vi "Event Structure String Replace Space 5.vi"() -> ()   [LabVIEW 2020]
panel:
  out "length":i32
  in  "String":string
  in  "Stop":bool
  # "Event Structure String : Replace Space"
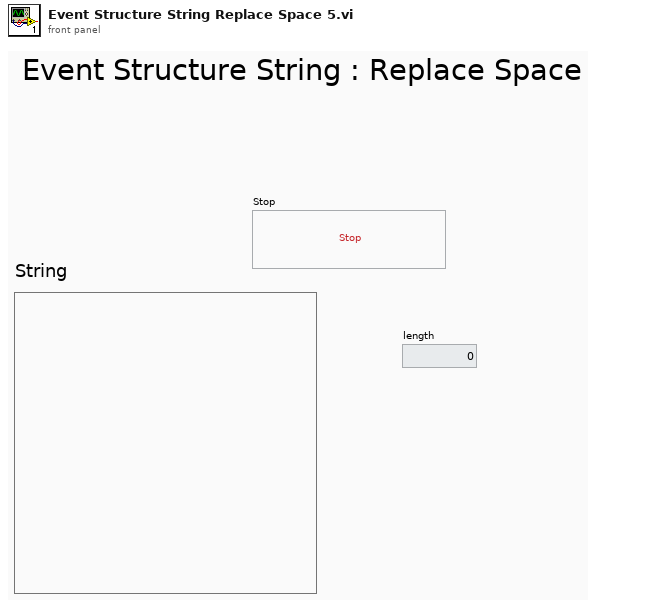
[diagram p1: front panel]
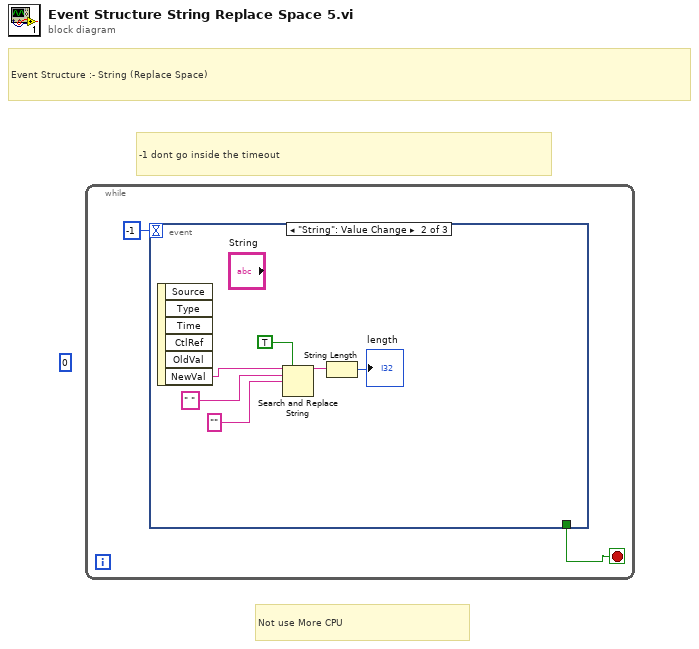
[diagram p0: block diagram]
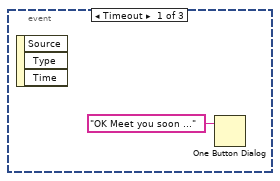
[diagram p2: hidden frame]
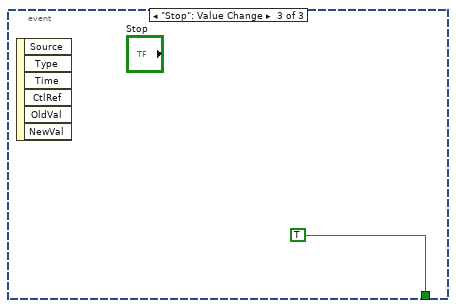
[diagram p3: hidden frame]
diagram:
  (unwired) 0
  # "Not use More CPU"
  # "-1 dont go inside the timeout"
  # "Event Structure :- String (Replace Space)"
  n1 = while {
    stop <- w1 stop-if-true
    n2 = event shown="[1] \"String\": Value Change" {
      selector: _ -> [_ _ _]
      dyn-events: _ -> [_ _ _]
      timeout: -1 -> [_ _ _]
      tunnel: [_ _ TRUE] -> w1
      event Timeout {
        n3 = event-data() -> ()  [unwired: 1 in, 3 out]
        n4 = One Button Dialog(message="OK Meet you soon ...") -> ()  [unwired: 1 in, 1 out]
      }
      event "String": Value Change {
        n5 = event-data() -> ("NewVal"=w9:string)  [unwired: 1 in, 5 out]
        n6 = Search and Replace String(replace all?=TRUE ("replace all? (F)"), input string=w9, search string=" ", replace string="" ("replace string (\"\")")) -> (result string=w6:string)  [unwired: 4 in, 3 out]
        n7 = String Length(string=w6) -> (length=→"length":i32)
      }
      event "Stop": Value Change {
        n8 = event-data() -> ()  [unwired: 1 in, 6 out]
      }
    }
  }
